vi "test.ingest_parquet.vi"   [LabVIEW 2020]
uses:
  datasources/dataset/dataset.lvclass
  nominal types/labels/labels.lvclass
  nominal types/properties/properties.lvclass
  datasources/dataset/dataset.lvclass/dataset.ctl
  Nominal Client/Nominal Client.lvclass/Nominal Client.ctl
  nominal types/workspace/workspace.lvclass/workspace.ctl
  81c5314d-0c17-4e40-9591-806fc92e59be.vi
  40e2c779-94f0-4ff6-913c-6196809b7e71.vi
  datasources/dataset/datasetName.set.vi
  Nominal Client/private_data.set.vi
  nominal types/workspace/id.get.vi
  nominal types/workspace/rid.get.vi
  <vilib>/AdvancedString/1D String Array to Delimited String.vi
  Nominal Client/workspace.set.vi
  datasources/gcs/gcs.lvclass
  C:/code/labview-client/lv_src/datasources/source/source.lvclass
  datasources/s3/s3.lvclass
  datasources/source/create_s3.vi
  datasources/target/create_from_existing.vi
  datasources/source/create_gcs.vi
  <vilib>/Utility/file.llb/Application Directory.vi
  <vilib>/Utility/error.llb/Error Cluster From Error Code.vi
  Nominal Client/Palette Items/who_am_i.vi
  datasources/target/create_new.vi
  ts.iso8601/build.iso8601.vi
  ts.relative/build.relative.vi
  Nominal Client/ingest_parquet.vi
  Nominal Client/workspace_cache.get_from_rid.vi
  Nominal Client/workspace_cache.get.vi
  User/User.lvclass
  Nominal Client/Nominal Client.lvclass
  nominal types/workspace/workspace.lvclass
  submodules/reqwest-labview/lv-src/reqwest/reqwest.lvclass
  timestampMetadata/timestampMetadata.lvclass
  datasources/target/target.lvclass
  datasources/source/source.lvclass
  nominal types/channelConfig/channelConfig.lvclass
  ts.iso8601/ts.iso8601.lvclass
  ts.relative/ts.relative.lvclass
  C:/code/labview-client/lv_src/datasources/payload/payload.lvclass
  C:/code/labview-client/lv_src/datasources/s3/s3.lvclass
  C:/code/labview-client/lv_src/datasources/gcs/gcs.lvclass
types:
  T1 = cluster{"channelPrefix":string, "tagKeysFromColumns":string[], "tagColums":map{string, string}, "additionalFileTags":map{string, string}, "isArchive?":bool}
  T2 = cluster{"channelPrefix":string, "tagKeysFromColumns":refnum<class "labels.lvclass">, "tagColums":refnum<class "properties.lvclass">, "additionalFileTags":refnum<class "properties.lvclass">, "isArchive":bool}
  T3 = enum16{"DAYS", "HOURS", "MINUTES", "SECONDS", "MILLISECONDS", "MICROSECONDS", "NANOSECONDS", "PICOSECONDS"}
  T4 = cluster{"dataset":refnum<class "dataset.lvclass">, "channelConfig":refnum<class "channelConfig.lvclass">}
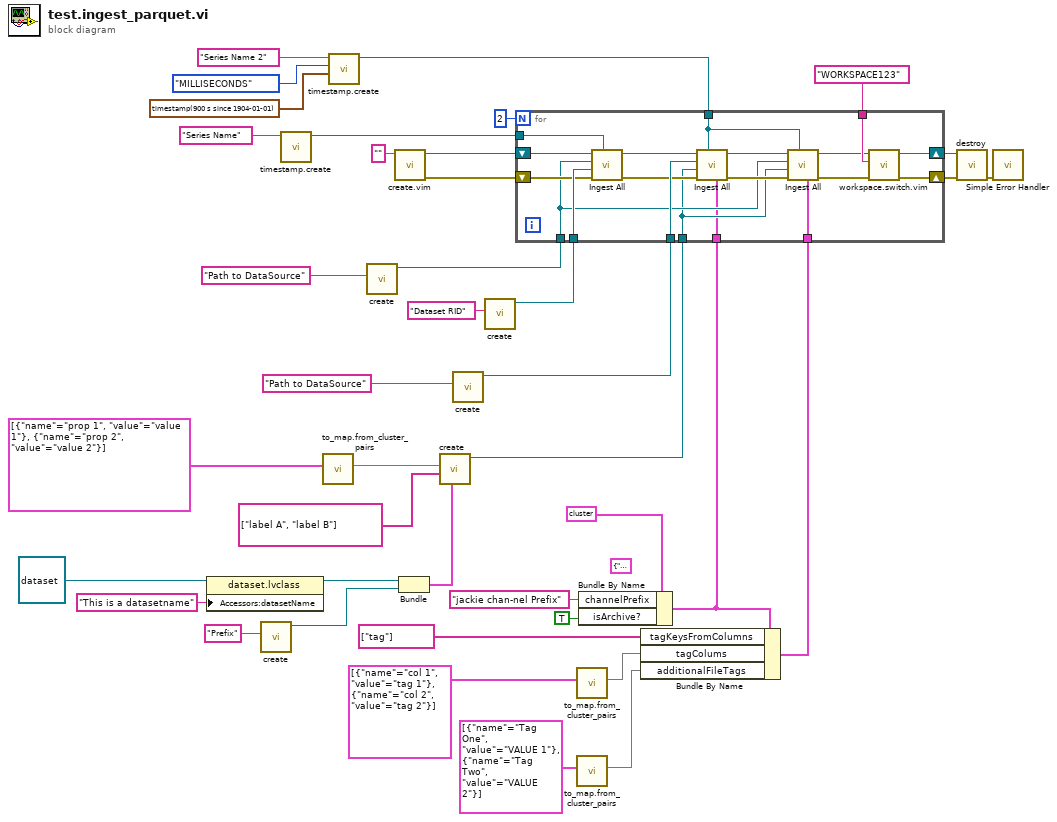
[diagram p0: block diagram]
diagram:
  (unwired) T2 {"channelPrefix"="", "tagKeysFromColumns"=refnum, "tagColums"=refnum, "additionalFileTags"=refnum, "isArchive"=FALSE} ("input cluster")
  n1 = property class="dataset.lvclass"(reference=refnum<class "dataset.lvclass"> refnum ("dataset"), "Accessors:datasetName"="This is a datasetname" ("datasetName")) -> (reference out=w32:refnum<class "dataset.lvclass">)  [unwired: 1 in, 1 out]
  n2 = call "create.vi"("prefixTreeDelimiter"="Prefix") -> ("channelConfig"=w10:refnum<class "channelConfig.lvclass">)  [unwired: 10 in]
  n3 = call-poly "timestamp.create.vi"("seriesName"="Series Name") -> ("Timestamp Metadata"=w30:refnum<class "timestampMetadata.lvclass">)  [unwired: 10 in]
  n4 = call "to_map.from_cluster_pairs.vi"("properties (cluster pairs)"=cluster{"name":string, "value":string}[] [{"name"="prop 1", "value"="value 1"}, {"name"="prop 2", "value"="value 2"}] ("properties")) -> ("properties (map)"=w7:map{string, string})  [unwired: 10 in]
  n5 = call-poly "timestamp.create.vi"("Offset"=timestamp(900 s since 1904-01-01), "Time Unit"=T3."MILLISECONDS", "Time Series Name"="Series Name 2" ("seriesName")) -> ("Timestamp Metadata"=w27:refnum<class "timestampMetadata.lvclass">)  [unwired: 8 in]
  n6 = call-poly "create.vi"("Path"="Path to DataSource") -> ("source"=w12:refnum<class "s3.lvclass">)  [unwired: 10 in]
  n7 = call "create.vim"("API Token (string or path)"="") -> ("error out"=w36:errorcluster, "Nominal Client"=w37:refnum<class "Nominal Client.lvclass">)  [unwired: 8 in, 1 out]
  n8 = Bundle("dataset"=w32, "channelConfig"=w10) -> (w17:T4)  [unwired: 1 in]
  n9 = call-poly "create.vi"("Optional"=w17, "Labels"=string[] ["label A", "label B"] ("labels"), "Properties"=w7) -> ("New Target"=w16:refnum<class "target.lvclass">)  [unwired: 8 in]
  n10 = call-poly "create.vi"("Path"="Path to DataSource") -> ("source"=w15:refnum<class "gcs.lvclass">)  [unwired: 10 in]
  n11 = call-poly "create.vi"("dataset RID"="Dataset RID" ("RID")) -> ("Existing Target"=w18:refnum<class "target.lvclass">)  [unwired: 10 in]
  n12 = call "to_map.from_cluster_pairs.vi"("properties (cluster pairs)"=cluster{"name":string, "value":string}[] [{"name"="col 1", "value"="tag 1"}, {"name"="col 2", "value"="tag 2"}] ("properties")) -> ("properties (map)"=w3:map{string, string})  [unwired: 10 in]
  n13 = call "to_map.from_cluster_pairs.vi"("properties (cluster pairs)"=cluster{"name":string, "value":string}[] [{"name"="Tag One", "value"="VALUE 1"}, {"name"="Tag Two", "value"="VALUE 2"}] ("properties")) -> ("properties (map)"=w2:map{string, string})  [unwired: 10 in]
  n14 = Bundle By Name(cluster=T1 {"channelPrefix"="", "tagKeysFromColumns"=[], "tagColums"={}, "additionalFileTags"={}, "isArchive?"=FALSE} ("optional"), "channelPrefix"="jackie chan-nel Prefix", "isArchive?"=TRUE ("isArchive")) -> (w22:T1)
  n15 = Bundle By Name(cluster=w22, "tagKeysFromColumns"=string[] ["tag"] ("labels"), "tagColums"=w3, "additionalFileTags"=w2) -> (w21:T1)
  n16 = for {
    N: 2 -> [_]
    tunnel: w18 -> [w59]
    tunnel: w12 -> [w46]
    tunnel: w15 -> [w58]
    tunnel: w16 -> [w45]
    shift-right: [w53] -> w38
    shift-left: w36 -> [w55]
    shift-right: [w52] -> w40
    shift-left: w37 -> [w54]
    tunnel: "WORKSPACE123" ("RID") -> [w51]
    tunnel: w30 -> [w44]
    tunnel: w27 -> [w43]
    tunnel: w22 -> [w42]
    tunnel: w21 -> [w41]
    n17 = call-poly "Ingest All.vi"("Timestamp Metadata"=w44, "error in"=w55, "Target"=w59, "Source"=w46, "Nominal Client in"=w54) -> ("error out"=w56:errorcluster, "Nominal Client out"=w57:refnum<class "Nominal Client.lvclass">)  [unwired: 3 in, 2 out]
    n18 = call-poly "Ingest All.vi"("optional"=w42, "Timestamp Metadata"=w43, "error in"=w56, "Target"=w45, "Source"=w58, "Nominal Client in"=w57) -> ("error out"=w50:errorcluster, "Nominal Client out"=w49:refnum<class "Nominal Client.lvclass">)  [unwired: 2 in, 2 out]
    n19 = call-poly "Ingest All.vi"("optional"=w41, "Timestamp Metadata"=w43, "error in"=w50, "Target"=w45, "Source"=w46, "Nominal Client in"=w49) -> ("error out"=w48:errorcluster, "Nominal Client out"=w47:refnum<class "Nominal Client.lvclass">)  [unwired: 2 in, 2 out]
    n20 = call "workspace.switch.vim"("error in"=w48, "Workspace (Object, RID, Path)"=w51, "Nominal Client in"=w47) -> ("error out"=w53:errorcluster, "Nominal Client out"=w52:refnum<class "Nominal Client.lvclass">)  [unwired: 7 in]
  }
  n21 = call "destroy.vi"("error in"=w38, "Nominal Client"=w40) -> ("error out"=w24:errorcluster)  [unwired: 9 in]
  n22 = call <vilib>:"Simple Error Handler.vi"("error in (no error)"=w24) -> ()  [unwired: 4 in, 5 out]
